vi "Append Message Header.vi"(11 "Message":string) -> (3 "Message with header":string)   [LabVIEW 2024, in "Ramses Framework.lvlib"]
doc: "Appends a 16bit message header to the beginning of a command string that will be sent over TCP/IP. Header is in the format;\n\n**XXXXXXXXXXXX**\n\nWhere X is a left justifed 64-bit integer with preceding zeros."
uses:
  Ramses Framework.lvlib
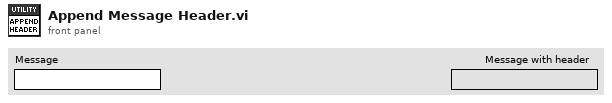
[diagram p1: front panel]
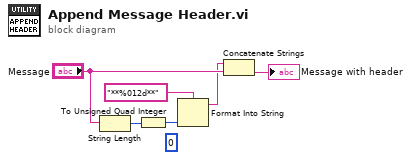
[diagram p0: block diagram]
diagram:
  (unwired) u64 0 ("unsigned 64bit integer")
  n1 = String Length(string="Message") -> (length=w5:i32)
  n2 = To Unsigned Quad Integer(1:w5) -> (0:w4:u64)
  n3 = Format Into String(format string="**%012d**", w4) -> (resulting string=w2:string)  [unwired: 2 in, 1 out]
  n4 = Concatenate Strings(w2, "Message") -> (→"Message with header":string)
